vi "Read.vi"(0 "TCS.lvclass in":refnum<class "TCS.lvclass">, 5 "error in (no error)":errorcluster, 6 "Unused":bool) -> (14 "TCS.lvclass out":refnum<class "TCS.lvclass">, 15 "I0":T1 {"Current" min=0.0}, 16 "I1":T1 {"Current" min=0.0}, 17 "I2":T1 {"Current" min=0.0}, 18 "I3":T1 {"Current" min=0.0}, 19 "error out":errorcluster)   [LabVIEW 2013, in "TCS.lvclass"]
uses:
  Lib.llb/TCS.lvclass
  Lib.llb/CS Data.ctl
  Lib.llb/CS.lvclass
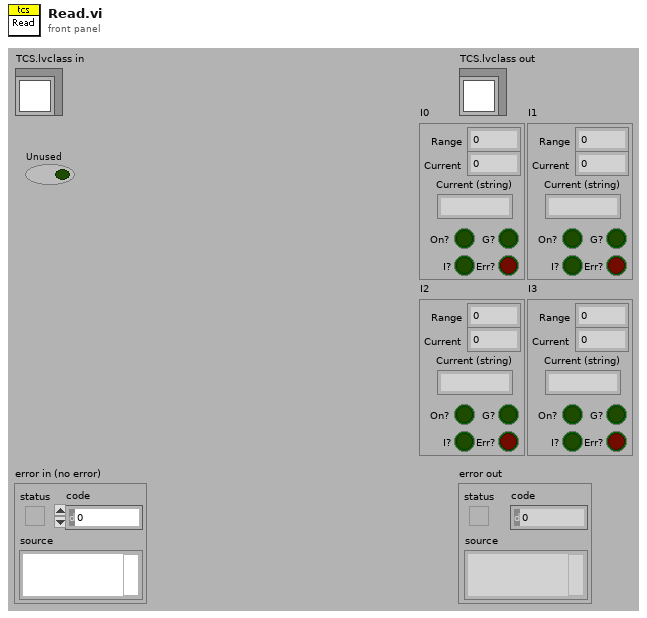
[diagram p1: front panel]
types:
  T1 = typedef "CS Data.ctl" = cluster{"Range":u8, "Current":dbl, "Current (string)":string, "On?":bool, "G?":bool, "I?":bool, "Err?":bool}
  T2 = cluster{"value (string)":string, "source on":bool, "source gated":bool, "c1":bool, "f1":bool}
  T3 = cluster{"value (string)":string, "source on":bool, "source gated":bool, "c2":bool, "f2":bool}
  T4 = cluster{"value (string)":string, "source on":bool, "source gated":bool, "c3":bool, "f3":bool}
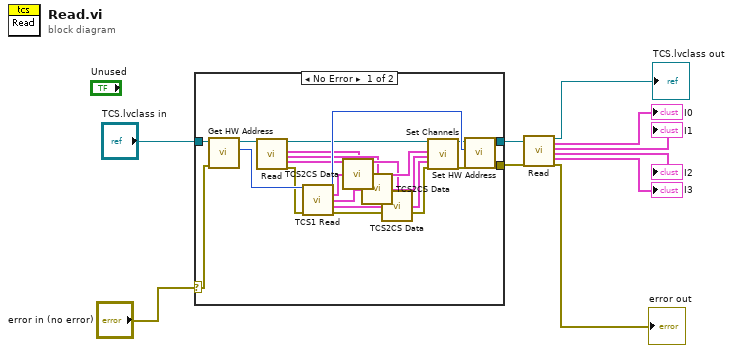
[diagram p0: block diagram]
diagram:
  n1 = case shown="No Error" "error in (no error)" {
    selector: "error in (no error)" -> [w30 w33]
    tunnel: "TCS.lvclass in" -> [w31 w32]
    tunnel: [w28 w33] -> w6
    tunnel: [w29 w32] -> w7
    frame No Error {
      n2 = call-dynamic "Get HW Address.vi"("error in (no error)"=w30, "CS.lvclass in"=w31) -> ("HW Address"=w27:u32, "CS.lvclass out"=w16:refnum<class "TCS.lvclass">)  [unwired: 7 in, 1 out]
      n3 = call-parent "Read.vi"("CS in"=w16) -> ("CS out"=w15:refnum<class "TCS.lvclass">, "I1"=w11:T1, "I2"=w12:T1, "I3"=w13:T1, "error out"=w14:errorcluster)  [unwired: 13 in, 1 out]
      n4 = call "TCS1 Read.vi"("port number in"=w27, "error in"=w14) -> ("port number out"=w26:u8, "CS1"=w20:T2, "CS2"=w21:T3, "CS3"=w22:T4, "error out"=w24:errorcluster)  [unwired: 9 in]
      n5 = call "TCS2CS Data.vi"("CS1"=w20, "I0"=w11) -> ("I0"=w17:T1)
      n6 = call "TCS2CS Data.vi"("CS1"=w21, "I0"=w12) -> ("I0"=w19:T1)
      n7 = call "TCS2CS Data.vi"("CS1"=w22, "I0"=w13) -> ("I0"=w18:T1)
      n8 = call-dynamic "Set Channels.vi"("CS.lvclass in"=w15, "I1"=w17, "I2"=w19, "I3"=w18, "error in (no error)"=w24) -> ("CS.lvclass out"=w25:refnum<class "TCS.lvclass">, "error out"=w23:errorcluster)  [unwired: 13 in]
      n9 = call-dynamic "Set HW Address.vi"("error in (no error)"=w23, "HW Address"=w26, "CS.lvclass in"=w25) -> ("error out"=w28:errorcluster, "CS.lvclass out"=w29:refnum<class "TCS.lvclass">)  [unwired: 7 in]
    }
    frame Error {
    }
  }
  n10 = call-parent "Read.vi"("CS in"=w7, "error in (no error)"=w6) -> ("CS out"=→"TCS.lvclass out":refnum<class "TCS.lvclass">, "I0"=→"I0":T1, "I1"=→"I1":T1, "I2"=→"I2":T1, "I3"=→"I3":T1, "error out"=→"error out":errorcluster)  [unwired: 12 in]
